vi "lab1_packet_formatter.vi"(8 "counter":i32, 9 "payload(bytes array)":u8[](array[numeric]), 11 "preamble(bytes array)":i16[](array[numeric])) -> (3 "bitstream":i16[](array[numeric]))   [LabVIEW 2014]
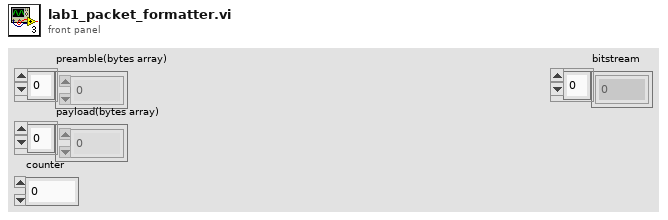
[diagram p1: front panel]
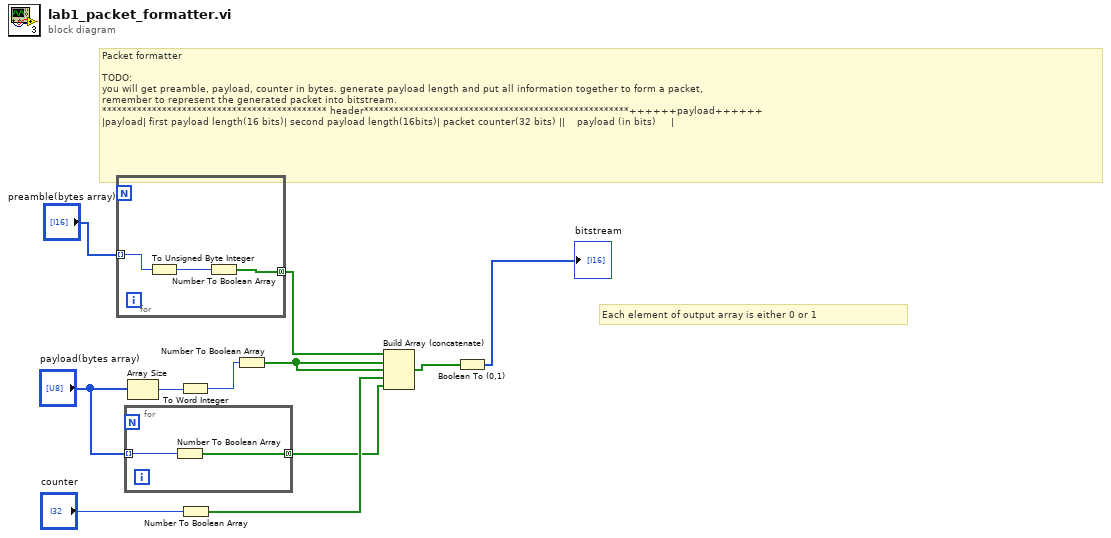
[diagram p0: block diagram]
diagram:
  # "Each element of output array is either 0 or 1"
  # "Packet formatter\n\nTODO: \nyou will get preamble, payload, counter in bytes. generate payload length and put all information together to form a packet, \nremember to represent the generated packet into bitstream. \n********************************************* header*****************************************************++++++payload++++++                  \n|payload| first payload length(16 bits)| second payload length(16bits)| packet counter(32 bits) ||    payload (in bits)     |"
  n1 = for {
    tunnel: "preamble(bytes array)" -> [w14] mode=indexing
    tunnel: [w13] -> w9 mode=concatenating
    n2 = To Unsigned Byte Integer(number=w14) -> (unsigned 8bit integer=w12:u8)
    n3 = Number To Boolean Array(number=w12) -> (Boolean array=w13:bool[])
  }
  n4 = for {
    tunnel: "payload(bytes array)" -> [w16] mode=indexing
    tunnel: [w15] -> w1 mode=concatenating
    n5 = Number To Boolean Array(number=w16) -> (Boolean array=w15:bool[])
  }
  n6 = Array Size(array="payload(bytes array)") -> (size(s)=w11:i32)
  n7 = To Word Integer(number=w11) -> (16bit integer=w8:i16)
  n8 = Number To Boolean Array(number="counter") -> (Boolean array=w5:bool[])
  n9 = Number To Boolean Array(number=w8) -> (Boolean array=w7:bool[])
  n10 = Build Array (concatenate)(w9, w7, w7, w5, w1) -> (w3:bool[])
  n11 = Boolean To (0,1)(Boolean=w3) -> (0, 1=→"bitstream":i16[])
